vi "AlliGator Use Phasor Plot UC-Segment Intersections as References.vi"(8 "Error In":errorcluster, 9 "Phasor Frequency":dbl[unit], 11 "Image Points":T2[](array[typedef])) -> (0 "error out":errorcluster, 1 "Point 2":T1, 2 "Point 1":T1)   [LabVIEW 2021, in "AlliGator Phasor Plot.lvlib"]
doc: "Defines the references as the intersection of the user-drawn segment and the UC in the Phasor Plot image."
uses:
  AlliGator Phasor Plot.lvlib
  Image/Image Point.ctl
  Phasor/Phasor (g, s).ctl
  AlliGator Phasor Ratio.lvlib
  Phasor/Phasor.lvlib
  Image/Image.lvlib
panel:
  # "see the AlliGator License on the block diagram (Ctrl+E or Window:Show Block Diagram)"
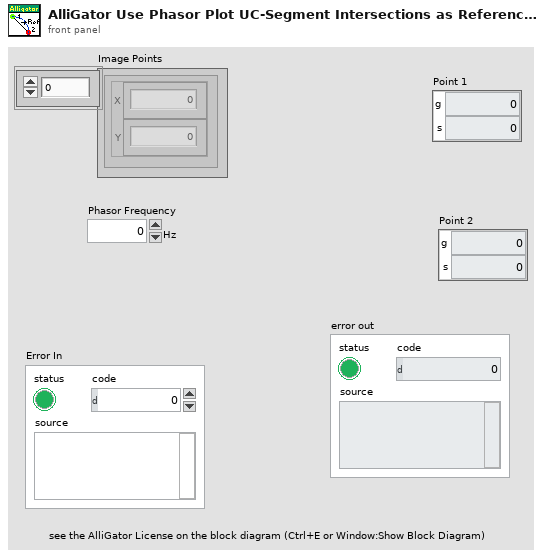
[diagram p1: front panel]
types:
  T1 = typedef "Phasor.lvlib/Phasor (g, s).ctl" = cluster{"g":dbl, "s":dbl}
  T2 = typedef "Image.lvlib/Image Point.ctl" = cluster{"X":i32, "Y":i32}
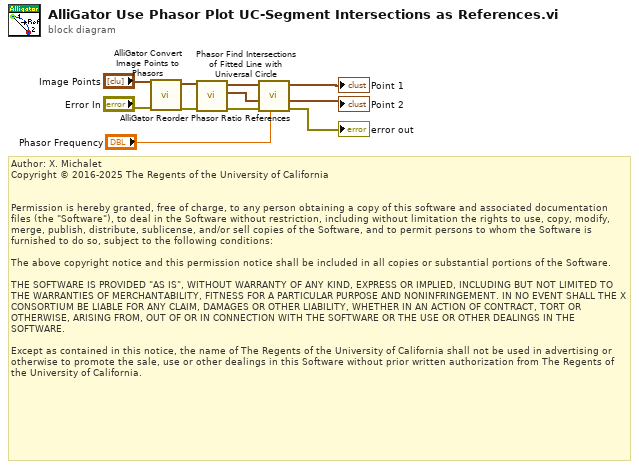
[diagram p0: block diagram]
diagram:
  # "Author: X. Michalet\nCopyright © 2016-2025 The Regents of the University of California\n \n\nPermission is hereby granted, free of charge, to any person obtaining a copy of this software and associated documentation files (the \"Software\"), to deal in the Software without restriction, including without limitation the rights to use, copy, modify, merge, publish, distribute, sublicense, and/or sell copies of the Software, and to permit persons to whom the Software is furnished to do so, subject to the following conditions:\n\nThe above copyright notice and this permission notice shall be included in all copies or substantial portions of the Software.\n\nTHE SOFTWARE IS PROVIDED \"AS IS\", WITHOUT WARRANTY OF ANY KIND, EXPRESS OR IMPLIED, INCLUDING BUT NOT LIMITED TO THE WARRANTIES OF MERCHANTABILITY, FITNESS FOR A PARTICULAR PURPOSE AND NONINFRINGEMENT. IN NO EVENT SHALL THE X CONSORTIUM BE LIABLE FOR ANY CLAIM, DAMAGES OR OTHER LIABILITY, WHETHER IN AN ACTION OF CONTRACT, TORT OR OTHERWISE, ARISING FROM, OUT OF OR IN CONNECTION WITH THE SOFTWARE OR THE USE OR OTHER DEALINGS IN THE SOFTWARE.\n\nExcept as contained in this notice, the name of The Regents of the University of California shall not be used in advertising or otherwise to promote the sale, use or other dealings in this Software without prior written authorization from The Regents of the University of California."
  n1 = call "AlliGator Convert Image Points to Phasors.vi"("Error In"="Error In", "Image Points"="Image Points") -> ("Error Out"=w8:errorcluster, "Phasors"=w9:T1[])  [unwired: 8 in]
  n2 = call "Phasor Find Intersections of Fitted Line with Universal Circle.vi"("Error In"=w8, "Phasor Array"=w9) -> ("Error Out"=w3:errorcluster, "Intersection 2"=w6:T1, "Intersection 1"=w7:T1)  [unwired: 7 in]
  n3 = call "AlliGator Reorder Phasor Ratio References.vi"("Phasor Frequency"="Phasor Frequency", "error in (no error)"=w3, "Phasor 2"=w6, "Phasor 1"=w7) -> ("error out"=→"error out":errorcluster, "Reference 2"=→"Point 2":T1, "Reference 1"=→"Point 1":T1)  [unwired: 3 in, 2 out]
